vi "Read Buffered Error.vi"(8 "error in":errorcluster, 9 "timeout in ms (0)":i32, 11 "Standard Engine Runtime in":refnum<class "Standard Engine Runtime.lvclass">) -> (0 "error out":errorcluster, 2 "Engine Error":errorcluster, 3 "Standard Engine Runtime out":refnum<class "Standard Engine Runtime.lvclass">)   [LabVIEW 2013, in "Standard Engine Runtime.lvclass"]
doc: "This method reads the engine's error queue. Use this method to get any error notifications from the engine."
uses:
  Standard Engine Runtime.lvclass
  Standard Engine Runtime.lvclass/Standard Engine Runtime.ctl
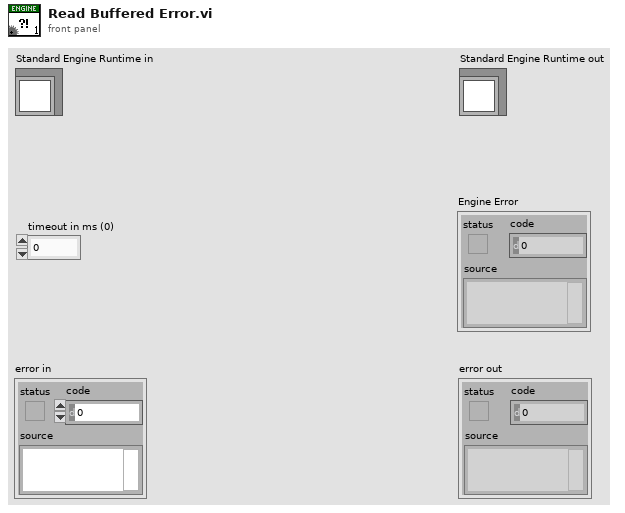
[diagram p1: front panel]
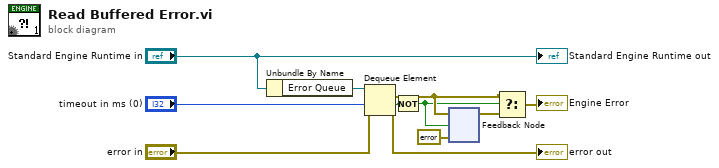
[diagram p0: block diagram]
diagram:
  n1 = Unbundle By Name("Standard Engine Runtime in") -> ("Error Queue"=w11:refnum<queue>)
  n2 = Dequeue Element(queue=w11, timeout in ms (-1)="timeout in ms (0)", error in (no error)="error in") -> (element=w4:errorcluster, timed out?=w6:bool, error out=→"error out":errorcluster)  [unwired: 1 out]
  n3 = Not(x=w6) -> (.not. x?=w3:bool)
  n4 = feedback-in #1(w4, w3) -> ()
  n5 = feedback #1(errorcluster {"status"=FALSE, "code"=0, "source"=""} ("error out")) -> (w5:errorcluster)
  n6 = Select(t=w4, s=w3, f=w5) -> (s? t:f=→"Engine Error":errorcluster)
  "Standard Engine Runtime out" <- "Standard Engine Runtime in"
